vi "get FPGA resource reservation info.vi"(8 "error in (no error)":errorcluster, 10 "Name in Bitfile":string, 11 "Item Ref in":T1 format="%.0x") -> (0 "error out":errorcluster, 1 "found?":bool, 2 "Reserver Node Ref":T1=18446744073709551615 format="%.0x", 3 "Item Ref out":T1 format="%.0x", 4 "notes":string, 5 "reserved?":bool)   [LabVIEW 2016, in "FPGA RM System Definition API.lvlib"]
uses:
  FPGA RM System Definition API.lvlib
  <vilib>/NI Veristand/Custom Device API/Custom Device Item Ref.ctl
  Shared/FPGA RM Shared API.lvlib
  <vilib>/NI VeriStand/Custom Device API/Custom Device API.lvlib
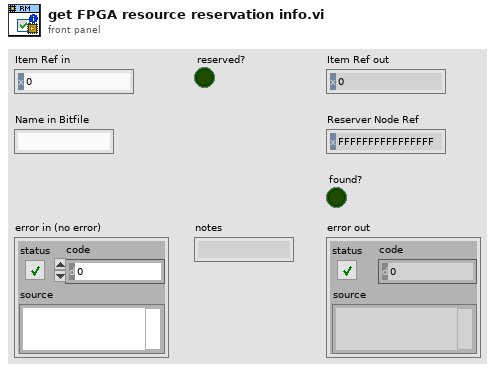
[diagram p1: front panel]
types:
  T1 = typedef "Custom Device API.lvlib/Custom Device Item Ref.ctl" = u64
  T2 = typedef "FPGA RM System Definition API.lvlib/fpga resource.ctl" = cluster{"name":string, "datatype":string, "channel type":T3, "value":variant, "notes":string}
  T3 = typedef "FPGA RM System Definition API.lvlib/Channel Type.ctl" = enum16{"Write Channel", "Read Channel", "Write Waveform", "Read Waveform"}
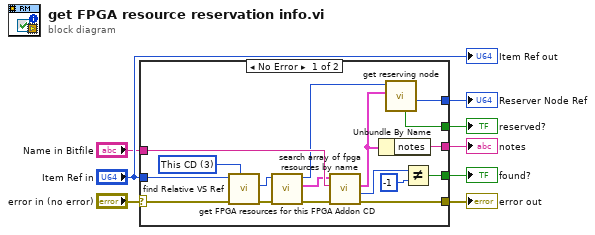
[diagram p0: block diagram]
diagram:
  n1 = case shown="No Error" "error in (no error)" {
    selector: "error in (no error)" -> [w22 w26]
    tunnel: [w16 w26] -> w7
    tunnel: "Item Ref in" -> [w23 _]
    tunnel: "Name in Bitfile" -> [w21 _]
    tunnel: [w18 _] -> w4
    tunnel: [w10 _] -> w3
    tunnel: [w17 _] -> w2
    tunnel: [w9 _] -> w1
    frame No Error {
      w25 = u16 3 items=["Targets", "Controller", "Custom Devices", "This CD", "This CD/Group", "This CD/Group/SubGroup"] ("Relative Type")
      n2 = call "find Relative VS Ref.vi"("Relative Type"=w25, "error in (no error)"=w22, "Item Ref in"=w23) -> ("error out"=w24:errorcluster, "Relative Item Ref Out"=w14:T1)  [unwired: 4 in, 3 out]
      n3 = call "get FPGA resources for this FPGA Addon CD.vi"("error in (no error)"=w24, "Item Ref in"=w14) -> ("error out"=w15:errorcluster, "fpga resources"=w13:T2[], "Item Ref out"=w12:T1)  [unwired: 6 in, 1 out]
      n4 = call "search array of fpga resources by name.vi"("error in (no error)"=w15, "Name in bitfile"=w21, "FPGA Resources in"=w13) -> ("error out"=w16:errorcluster, "index of element"=w20:i32, "FPGA Resource"=w11:T2)  [unwired: 6 in]
      n5 = Unbundle By Name(w11) -> ("notes"=w17:string)
      n6 = call "get reserving node.vi"("FPGA Resource"=w11, "Item Ref in"=w12) -> ("Dependent Node Ref"=w10:T1, "Found"=w9:bool)  [unwired: 6 in, 2 out]
      n7 = Not Equal?(x=w20, y=-1) -> (x != y?=w18:bool)
    }
    frame Error {
    }
  }
  "error out" <- w7
  "found?" <- w4
  "Reserver Node Ref" <- w3
  "notes" <- w2
  "reserved?" <- w1
  "Item Ref out" <- "Item Ref in"
